vi "PI-Mono-Power.vi"() -> ()   [LabVIEW 2009]
uses:
  <vilib>/Utility/file.llb/Write To Spreadsheet File (DBL).vi
  <vilib>/Analysis/NI_AALBase.lvlib
  <vilib>/DAQmx/create/channels.llb/DAQmx Create Channel (AI-Voltage-Basic).vi
  <vilib>/DAQmx/configure/timing.llb/DAQmx Timing (Sample Clock).vi
  <vilib>/DAQmx/read.llb/DAQmx Read (Analog 1D DBL 1Chan NSamp).vi
  <vilib>/Utility/file.llb/Read From Spreadsheet File (DBL).vi
panel:
  in  "Open Power Normalization Values Path":path
  in  "Normalize with file?":bool
  in  "Power Values Path":path
  out "Normalized Current":cluster{dbl[], dbl[]}(graph)
  in  "Save Current Path":path
  in  "Save Current?":bool
  out "Spectral Current":cluster{dbl[], dbl[]}(graph)
  in  "End Scan":bool
  out "Measuring Current":bool
  in  "Current":tag
  in  "Current Scan":bool
  in  "Exit":bool
  out "Scanning":bool
  in  "Scan Save Path":path
  in  "Save Power Scan?":bool
  out "Power Scan":cluster{dbl[], dbl[]}(graph)
  in  "Abort\n Scan":bool
  in  "Wavelength\n   Step Size":dbl=1.0 min=0.1 max=100.0
  in  "Starting\nWavelength":dbl=400.0 min=400.0 max=2500.0
  in  "Ending\nWavelength":dbl=500.0 min=451.0 max=2501.0
  in  "Step Time (sec)":dbl=1.0 min=0.1 max=10.0 step=0.1
  in  "Measurement Save Path":path
  in  "Save Measurement?":bool
  out "Power Measurement":dbl[](graph)
  out "Readout value":dbl format="%^#_9e"
  out "Readout string":string
  in  "Timeout [ms]":i32=1000
  out "New":bool
  out "ZeroValue":dbl
  out "RANG_Val":dbl
  out "RANG_lbl":string
  out "Rng":string
  out "AUTO?":bool
  in  "AUTO":bool=TRUE
  in  "Range":i16=1 min=1 max=6 step=1
  out "PM Error log":string
  in  "Beam\nDiameter (mm)":dbl=4.0 min=1.0 max=9.0 step=0.5
  in  "BWIn":u16(ring) caption="Bandwidth" items=["HIGH", "LOW"]
  in  "Averaging Rate":i32=300 min=33 max=5000 step=1
  in  "Zero?":bool
  in  "Stop Measurement":bool
  out "Incrementing Down":bool
  out "Changing Wavelength":bool
  out "Incrementing Up":bool
  in  "Increment":dbl=10.0 min=0.1 max=50.0
  in  "Target\nWavelength":dbl=400.0 min=400.0 max=3000.0
  out "Wavelength (nm)":dbl
  out "Turning Turret":bool
  out "Current Blaze":string caption="Grating Blaze"
  out "Grating Density":dbl
  out "Grating Index":i32
  in  "Select Grating Blaze":string(combo)
  out "error out":errorcluster
  in  "Measure Power":bool
  in  "Switch Turret":bool
  in  "Scan":bool
  in  "Increment Down":bool
  in  "Increment Up":bool
  in  "Change Wavelength":bool
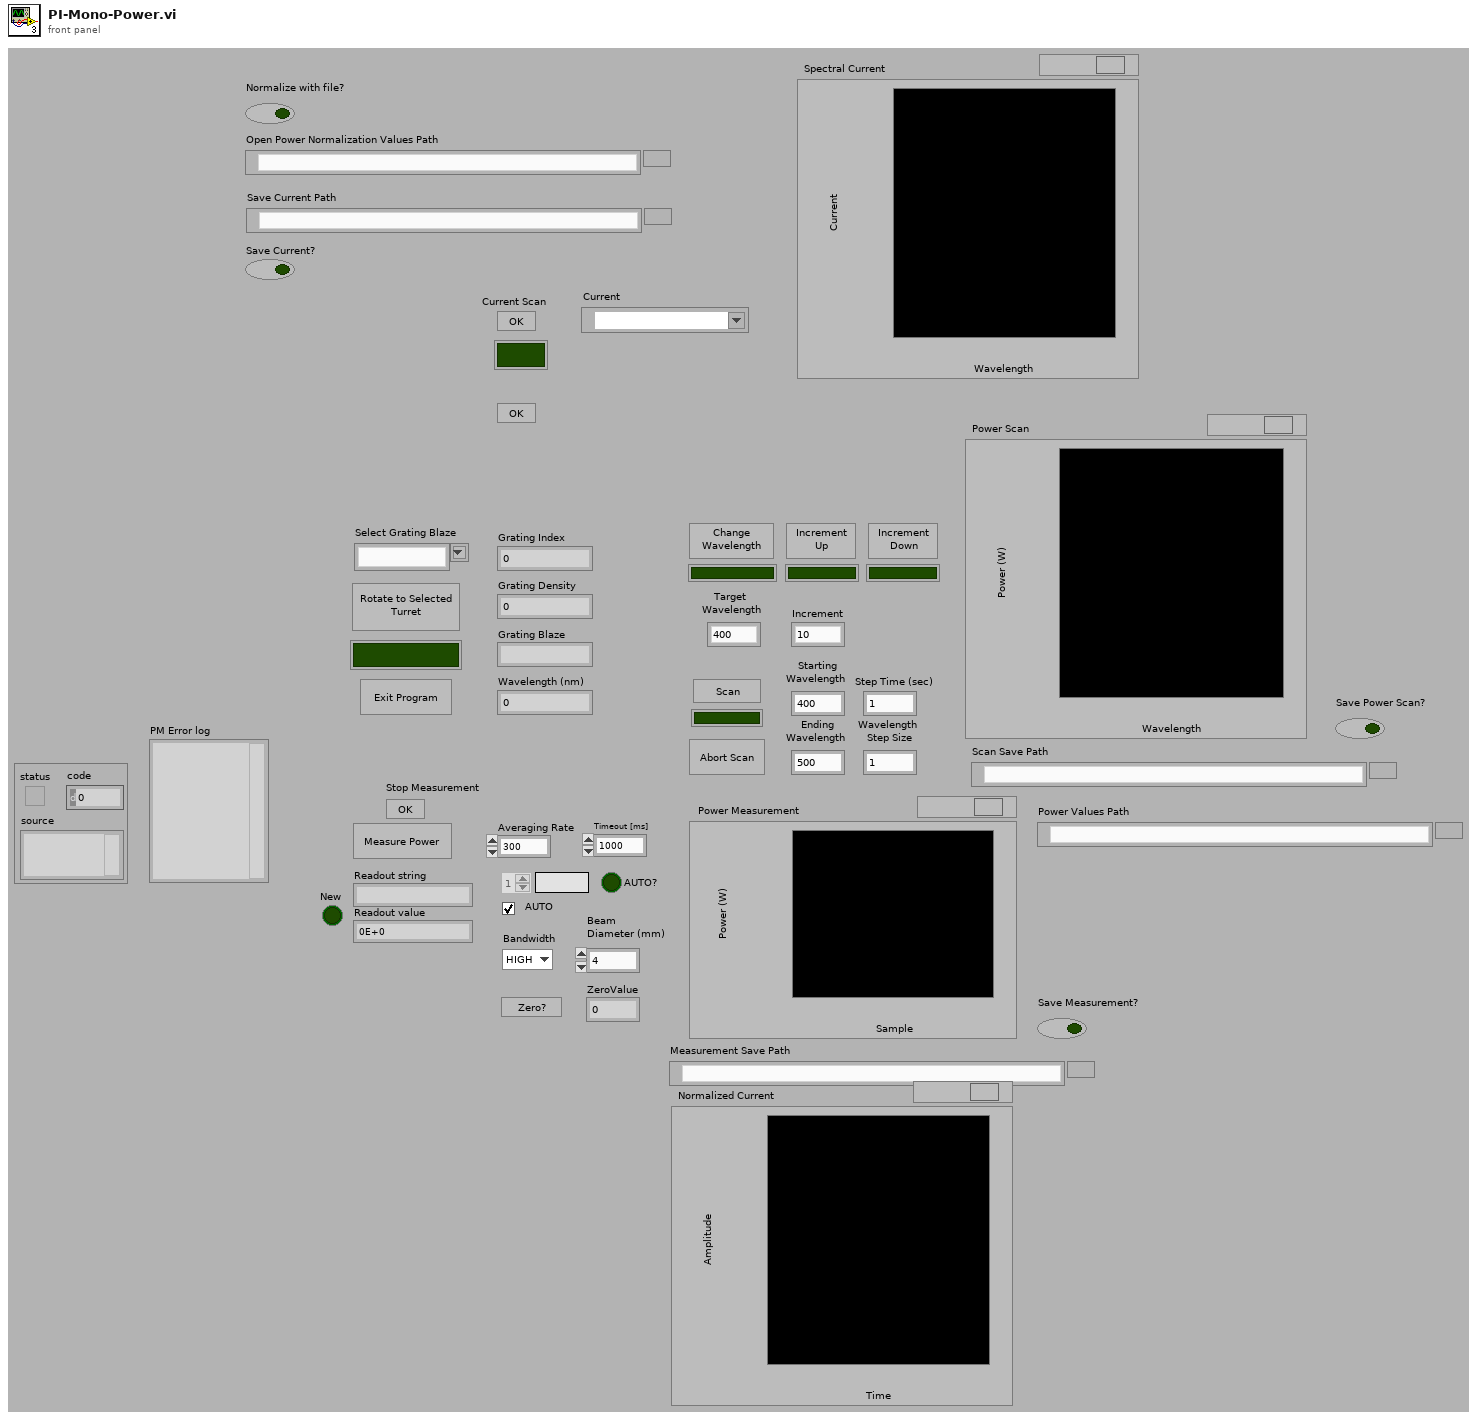
[diagram p1: front panel]
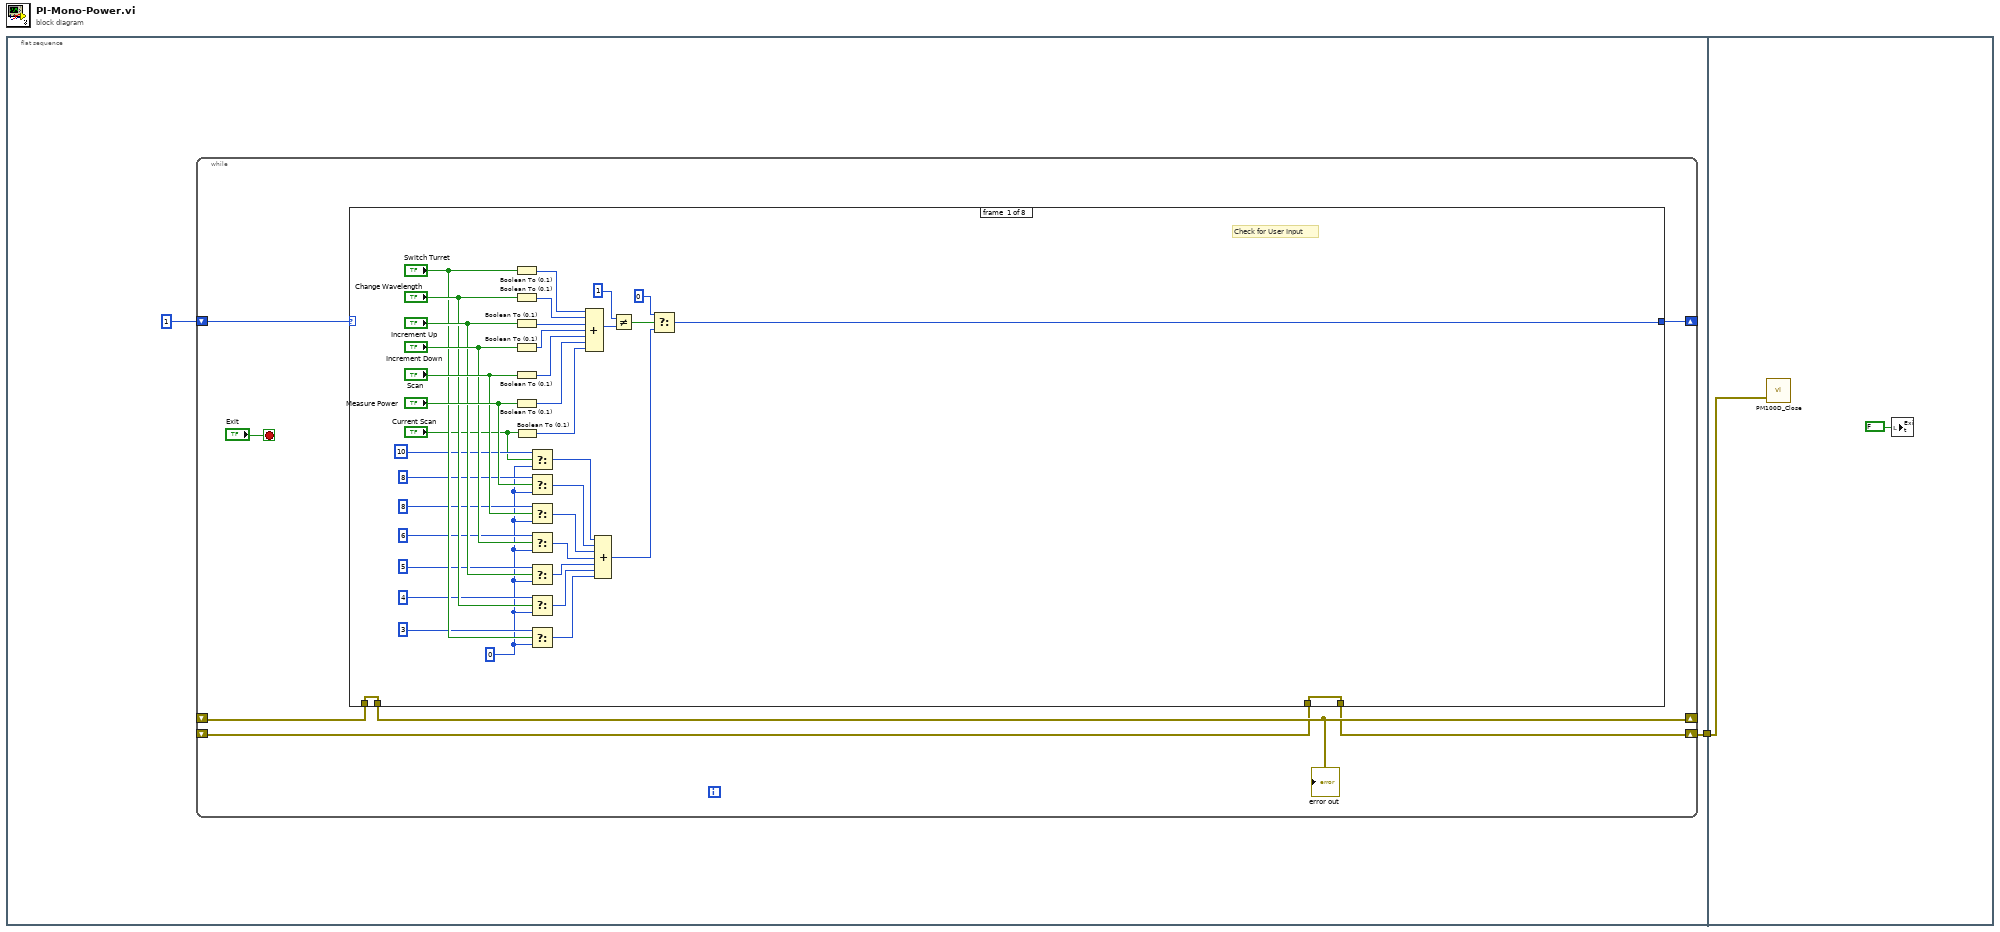
[diagram p0: block diagram]
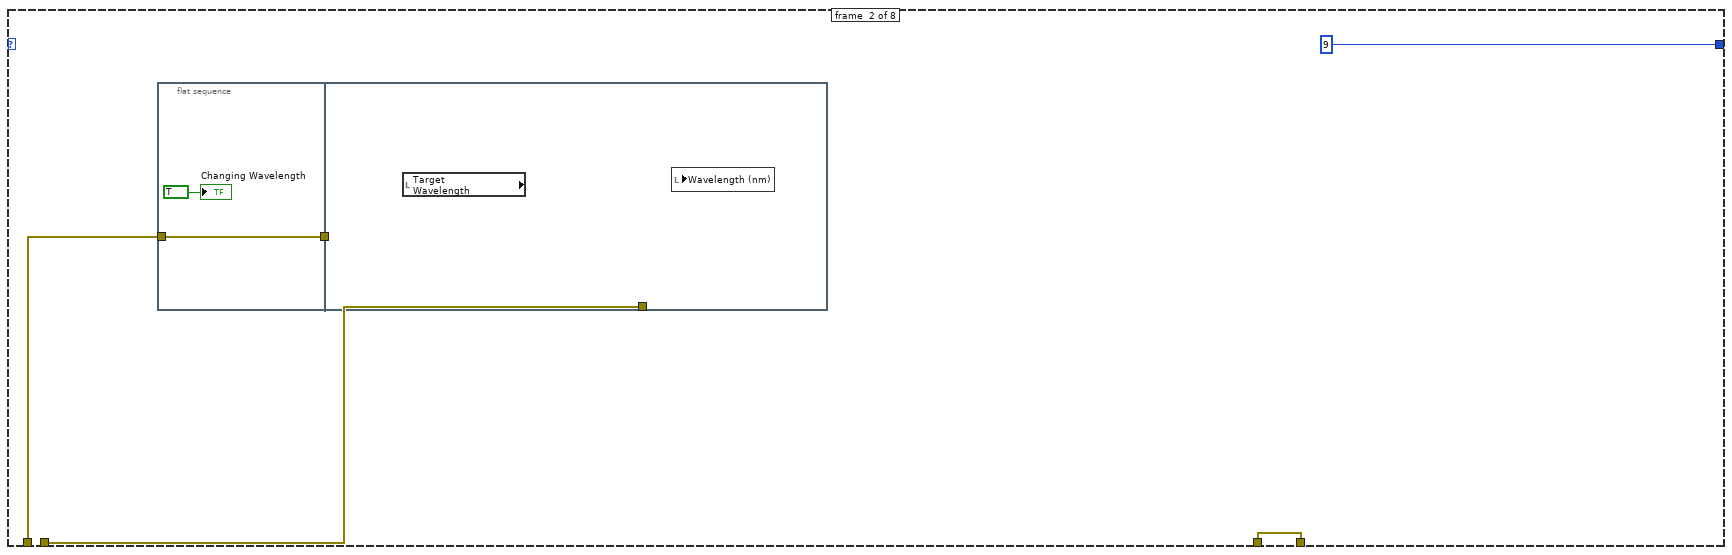
[diagram p2: hidden frame]
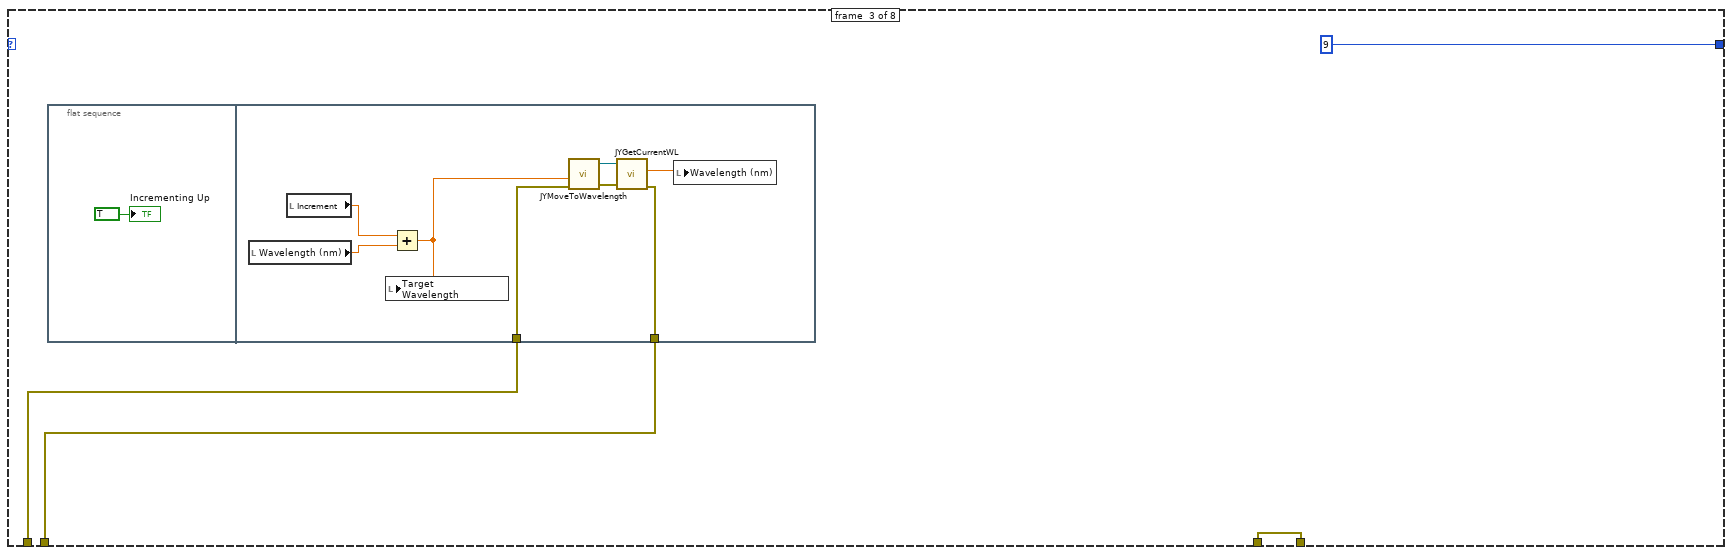
[diagram p3: hidden frame]
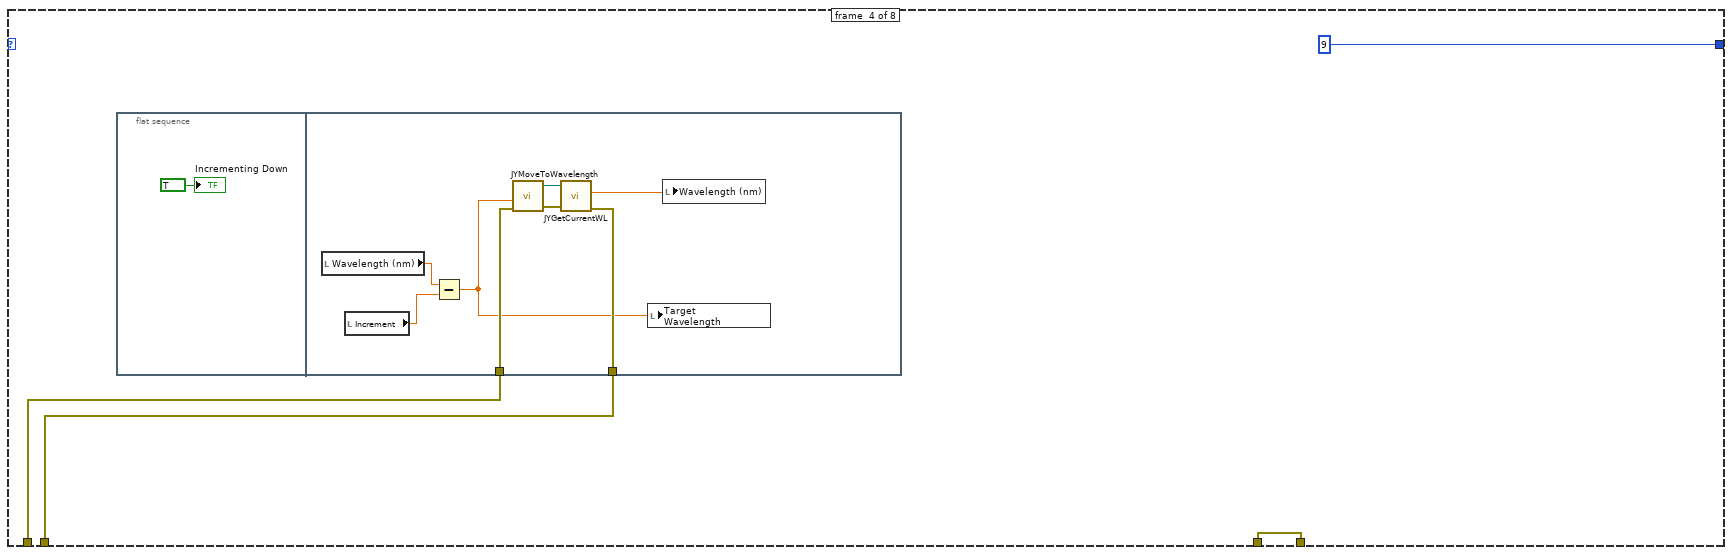
[diagram p4: hidden frame]
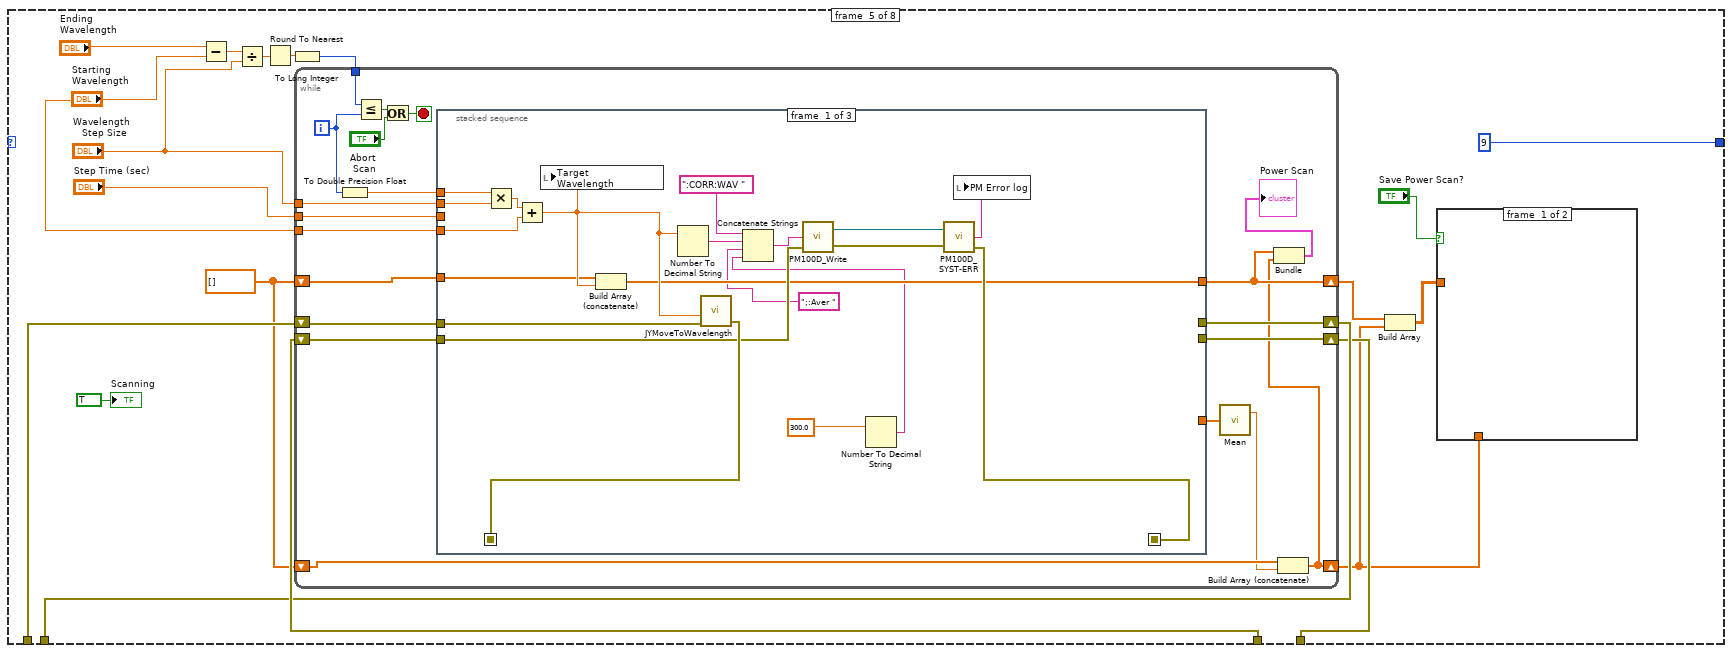
[diagram p5: hidden frame]
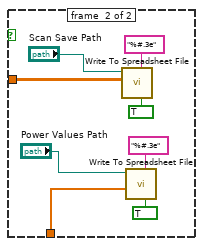
[diagram p6: hidden frame]
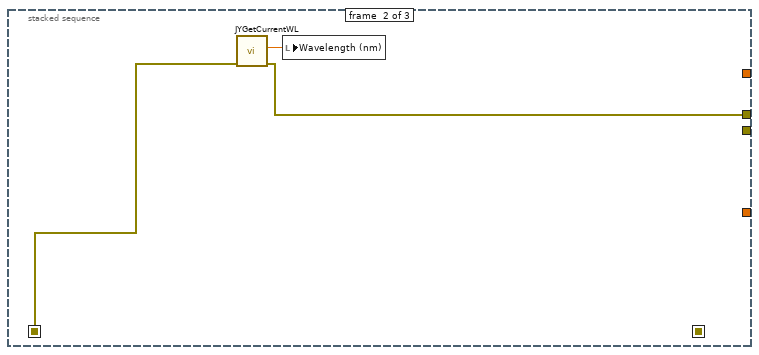
[diagram p7: hidden frame]
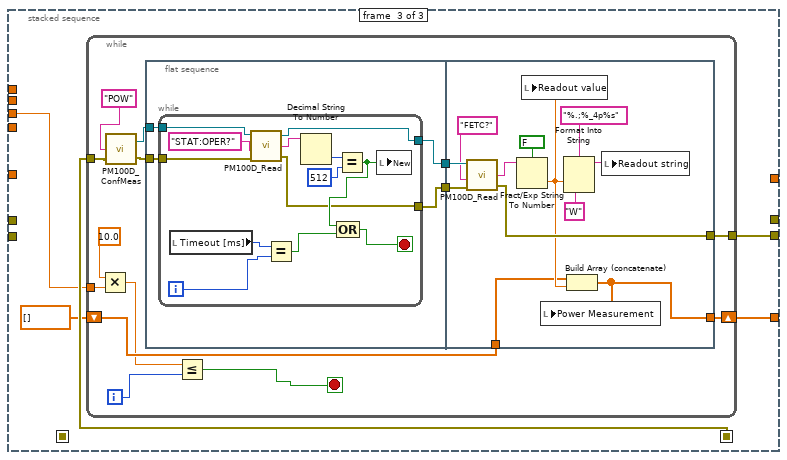
[diagram p8: hidden frame]
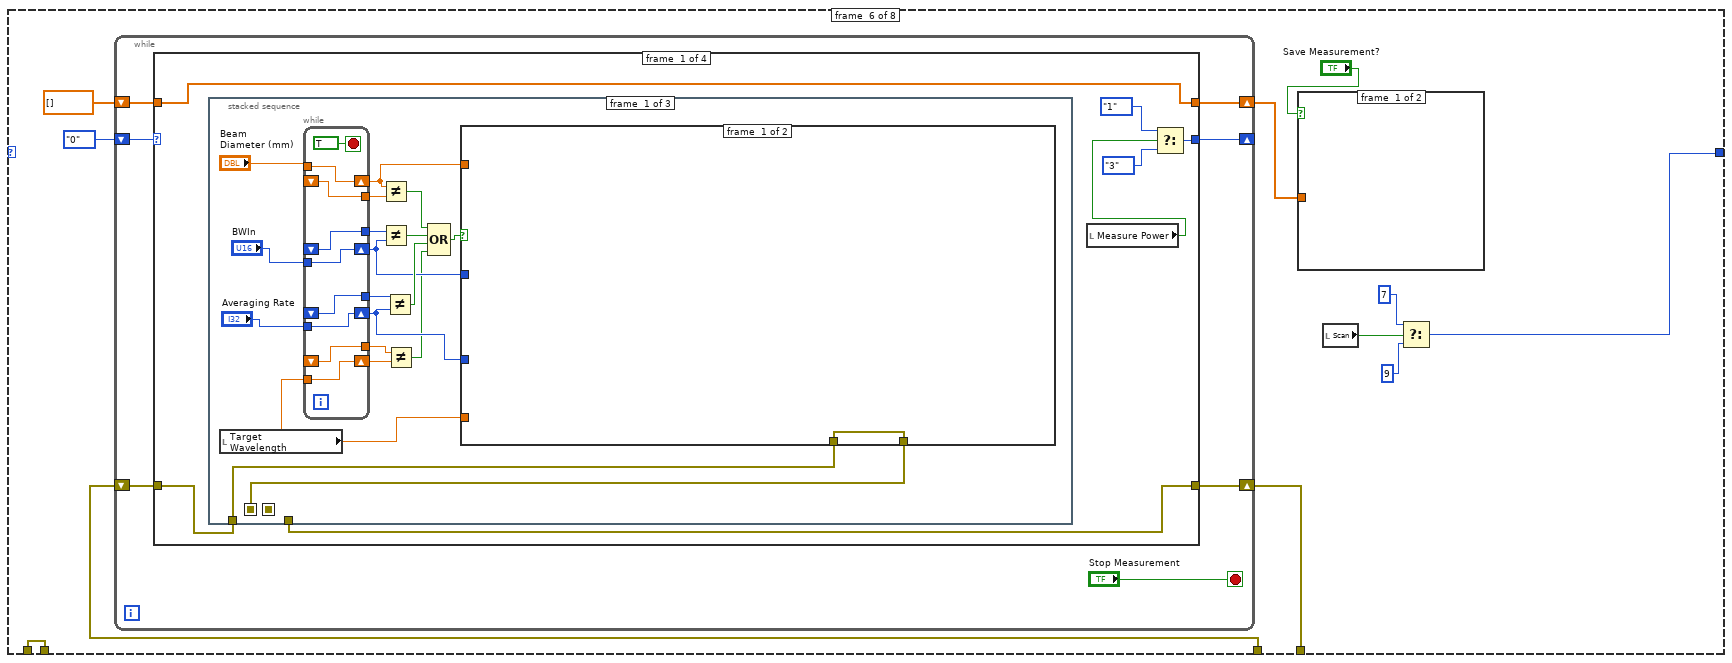
[diagram p9: hidden frame]
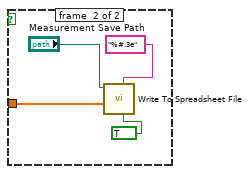
[diagram p10: hidden frame]
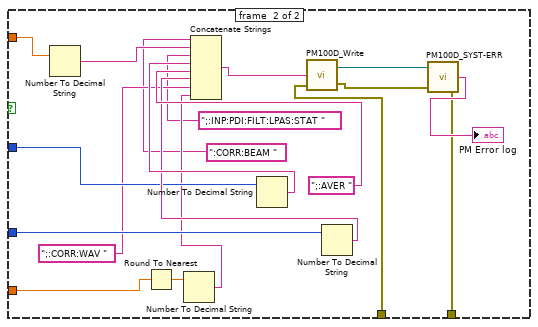
[diagram p11: hidden frame]
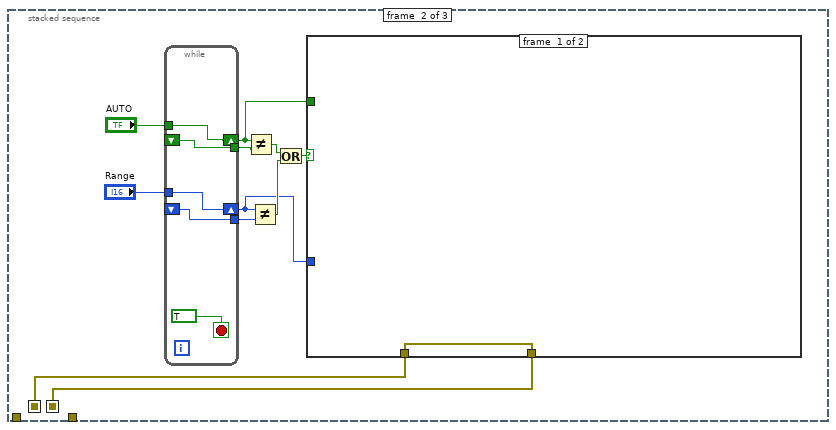
[diagram p12: hidden frame]
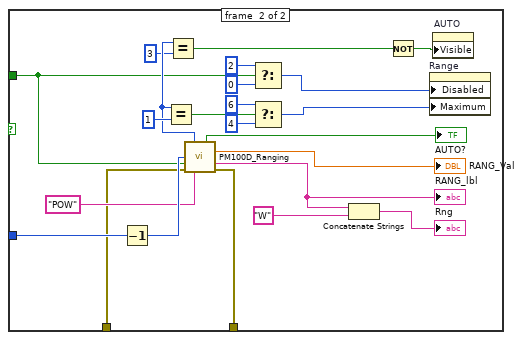
[diagram p13: hidden frame]
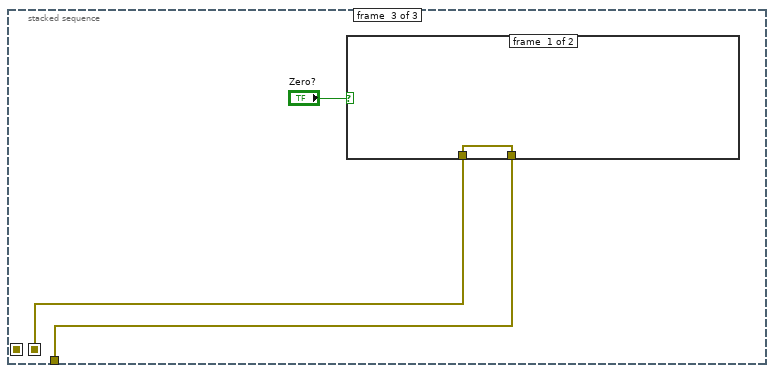
[diagram p14: hidden frame]
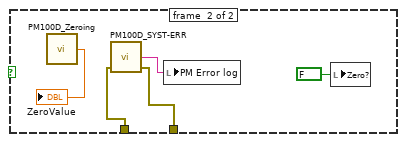
[diagram p15: hidden frame]
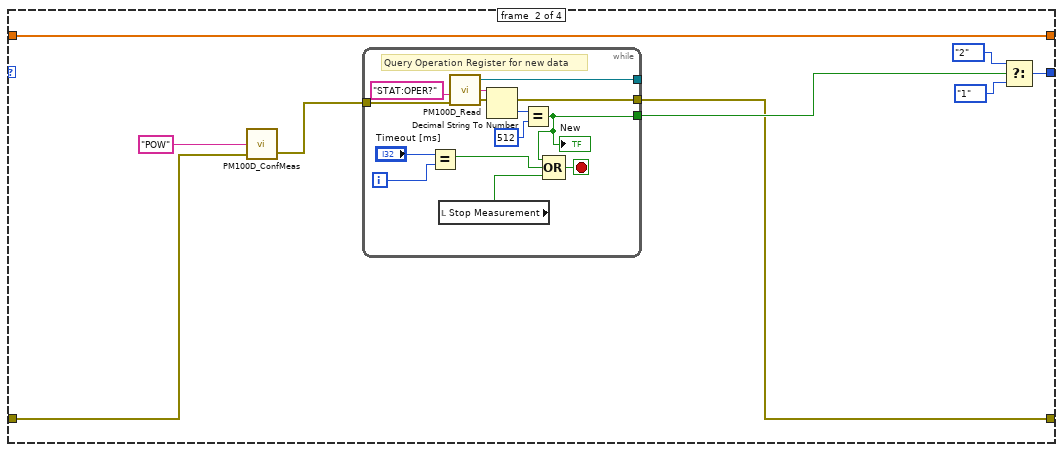
[diagram p16: hidden frame]
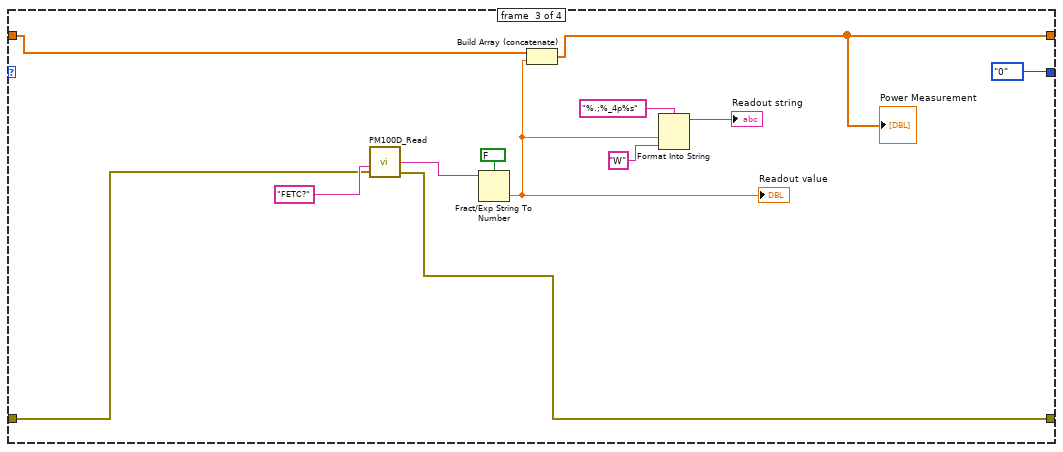
[diagram p17: hidden frame]
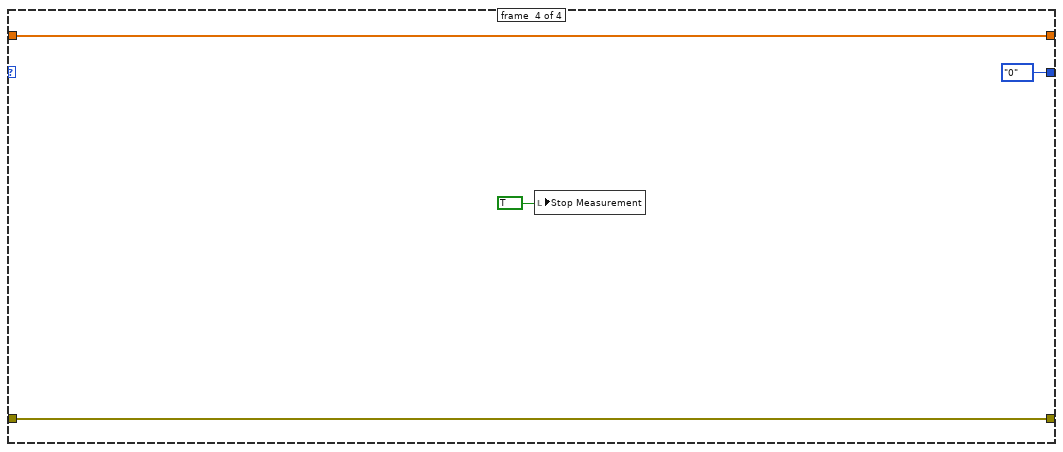
[diagram p18: hidden frame]
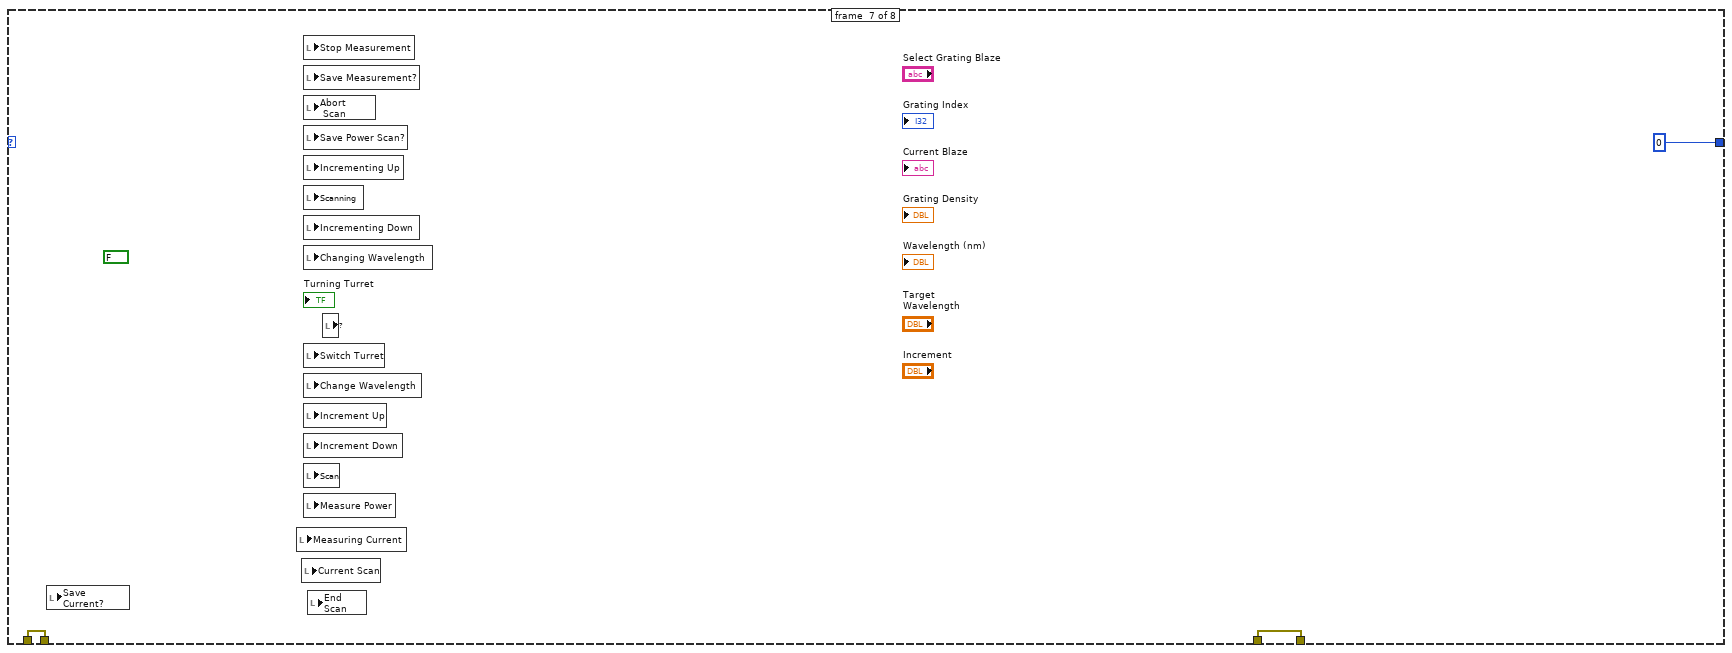
[diagram p19: hidden frame]
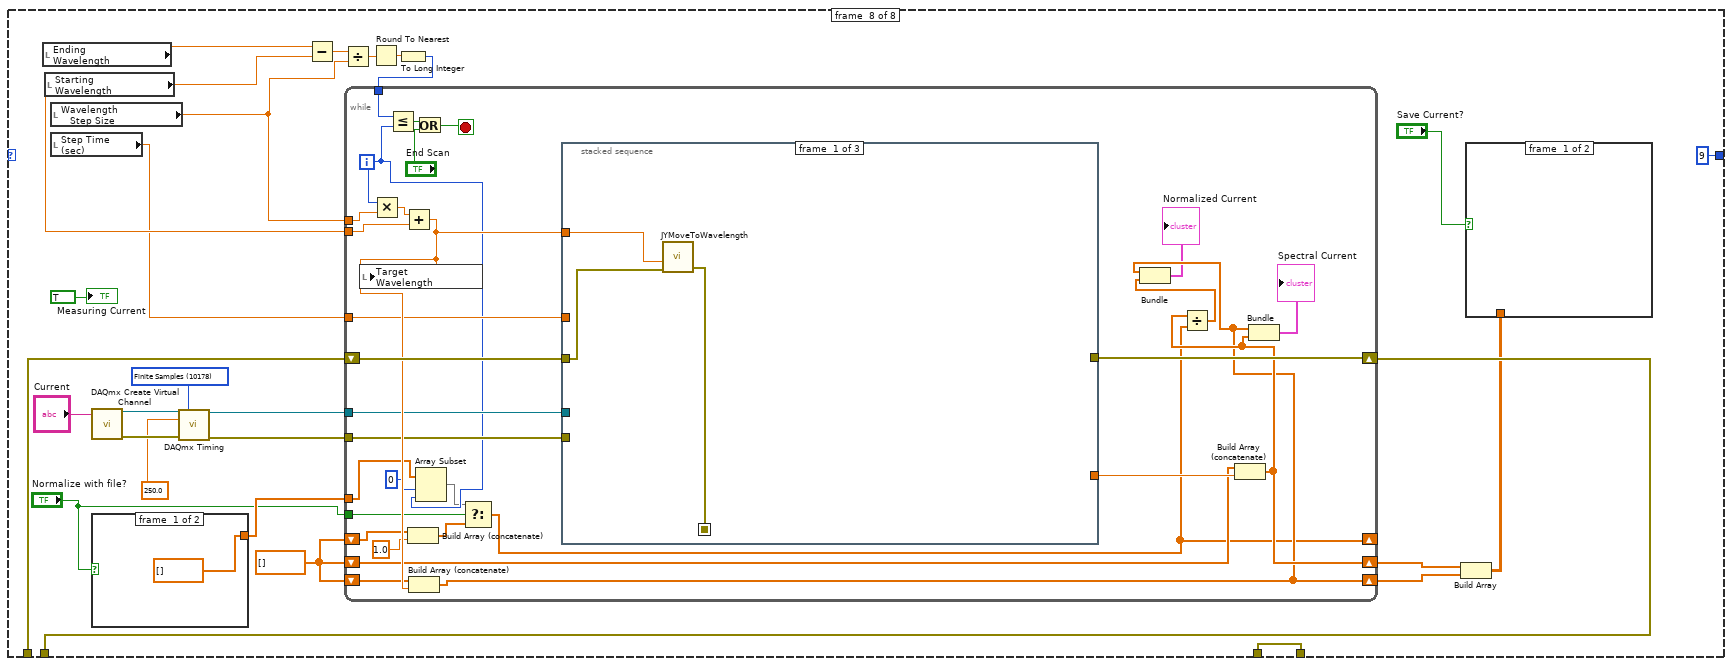
[diagram p20: hidden frame]
diagram:
  n1 = flat-sequence {
    tunnel: [w3] -> w1
    tunnel: w1 -> [w450]
    frame #0 {
      n2 = while {
        shift-right: [w10] -> _
        shift-left: 1 ("x") -> [w9]
        shift-right: [w7] -> _
        shift-left: _ -> [w8]
        shift-right: [w6] -> w3
        shift-left: _ -> [w5]
        stop <- "Exit" stop-if-true
        n3 = case shown="4" w9 {
          tunnel: [w19 9 ("x") 9 ("x") 9 ("x") 9 ("x") w199 0 ("x") 9 ("x")] -> w10
          tunnel: [w17 w50 w56 w70 w90 w209 w365 w382] -> w7
          tunnel: w8 -> [w17 w51 w57 w71 w92 w209 w365 w383]
          tunnel: [w16 w48 w55 w68 w89 w206 w364 w377] -> w6
          tunnel: w5 -> [w16 w48 w55 w68 w91 w207 w364 w377]
          frame #0 {
            w13 = 0 ("x")
            # "Check for User Input"
            n4 = Boolean To (0,1)(Boolean="Switch Turret") -> (0, 1=w47:i16)
            n5 = Boolean To (0,1)(Boolean="Change Wavelength") -> (0, 1=w46:i16)
            n6 = Boolean To (0,1)(Boolean="Increment Up") -> (0, 1=w45:i16)
            n7 = Boolean To (0,1)(Boolean="Increment Down") -> (0, 1=w44:i16)
            n8 = Boolean To (0,1)(Boolean="Scan") -> (0, 1=w43:i16)
            n9 = Boolean To (0,1)(Boolean="Measure Power") -> (0, 1=w42:i16)
            n10 = Boolean To (0,1)(Boolean="Current Scan") -> (0, 1=w15:i16)
            n11 = Select(t=10 ("x"), s="Current Scan", f=w13) -> (s? t:f=w14:i32)
            n12 = Select(t=8 ("x"), s="Measure Power", f=w13) -> (s? t:f=w33:i32)
            n13 = Select(t=8 ("x"), s="Scan", f=w13) -> (s? t:f=w32:i32)
            n14 = Select(t=6 ("x"), s="Increment Down", f=w13) -> (s? t:f=w31:i32)
            n15 = Select(t=5 ("x"), s="Increment Up", f=w13) -> (s? t:f=w30:i32)
            n16 = Select(t=4 ("x"), s="Change Wavelength", f=w13) -> (s? t:f=w29:i32)
            n17 = Select(t=3 ("x"), s="Switch Turret", f=w13) -> (s? t:f=w28:i32)
            n18 = Compound Arithmetic op=ADD(w47, w46, w45, w44, w43, w42, w15) -> (w41:i16)
            n19 = Compound Arithmetic op=ADD(w14, w33, w32, w31, w30, w29, w28) -> (w20:i32)
            n20 = Not Equal?(x=i16 1, y=w41) -> (x != y?=w27:bool)
            n21 = Select(t=0 ("x"), s=w27, f=w20) -> (s? t:f=w19:i32)
          }
          frame #1 {
            n22 = flat-sequence {
              tunnel: w51 -> [w54]
              tunnel: [w54] -> w49
              tunnel: [_] -> w50
              tunnel: w49 -> [_]
              frame #0 {
                "Changing Wavelength" <- TRUE
              }
              frame #1 {
                n23 = local read "Target\nWavelength"() -> ()  [unwired: 1 out]
                n24 = local read "Wavelength (nm)"() -> ()  [unwired: 1 in]
              }
            }
          }
          frame #2 {
            n25 = flat-sequence {
              tunnel: w57 -> [w65]
              tunnel: [w62] -> w56
              frame #0 {
                "Incrementing Up" <- TRUE
              }
              frame #1 {
                n26 = local read "Wavelength (nm)"() -> (w66:dbl)
                n27 = local read "Increment"() -> (w67:dbl)
                n28 = Add(x=w67, y=w66) -> (x+y=w61:dbl)
                n29 = local write "Target\nWavelength"(w61) -> ()
                n30 = call "JYMoveToWavelength.vi"("error in (no error)"=w65, "Target WL"=w61) -> ("error out"=w64:errorcluster, "Refnum Out"=w63:refnum<k7>)  [unwired: 2 in, 1 out]
                n31 = call "JYGetCurrentWL.vi"("error in (no error)"=w64, "JYMONOLib.IJYMonoReqd"=w63) -> ("error out"=w62:errorcluster, "Current WL"=w60:dbl)  [unwired: 6 in, 2 out]
                n32 = local write "Wavelength (nm)"(w60) -> ()
              }
            }
          }
          frame #3 {
            n33 = flat-sequence {
              tunnel: w71 -> [w76]
              tunnel: [w75] -> w70
              frame #0 {
                "Incrementing Down" <- TRUE
              }
              frame #1 {
                n34 = local read "Wavelength (nm)"() -> (w78:dbl)
                n35 = local read "Increment"() -> (w77:dbl)
                n36 = Subtract(x=w78, y=w77) -> (x-y=w74:dbl)
                n37 = call "JYMoveToWavelength.vi"("error in (no error)"=w76, "Target WL"=w74) -> ("error out"=w80:errorcluster, "Refnum Out"=w79:refnum<k7>)  [unwired: 2 in, 1 out]
                n38 = call "JYGetCurrentWL.vi"("error in (no error)"=w80, "JYMONOLib.IJYMonoReqd"=w79) -> ("error out"=w75:errorcluster, "Current WL"=w73:dbl)  [unwired: 6 in, 2 out]
                n39 = local write "Target\nWavelength"(w74) -> ()
                n40 = local write "Wavelength (nm)"(w73) -> ()
              }
            }
          }
          frame #4 {
            w88 = dbl[] []
            n41 = Subtract(x="Ending\nWavelength", y="Starting\nWavelength") -> (x-y=w97:dbl)
            n42 = Divide(x=w97, y="Wavelength\n   Step Size") -> (x/y=w83:dbl)
            n43 = Round To Nearest(number=w83) -> (nearest integer value=w82:dbl)
            n44 = To Long Integer(number=w82) -> (32bit integer=w96:i32)
            n45 = while {
              tunnel: w96 -> [w127]
              tunnel: "Wavelength\n   Step Size" -> [w123]
              tunnel: "Step Time (sec)" -> [w122]
              tunnel: "Starting\nWavelength" -> [w121]
              shift-right: [w110] -> w87
              shift-left: w88 -> [w116]
              shift-right: [w115] -> w90
              shift-left: w92 -> [w118]
              shift-right: [w114] -> w89
              shift-left: w91 -> [w117]
              shift-right: [w109] -> w81
              shift-left: w88 -> [w112]
              i -> [w120]
              stop <- w125 stop-if-true
              n46 = To Double Precision Float(number=w120) -> (double precision float=w119:dbl)
              n47 = Less Or Equal?(x=w127, y=w120) -> (x <= y?=w126:bool)
              n48 = Or(x=w126, y="Abort\n Scan") -> (x .or. y?=w125:bool)
              n49 = stacked-sequence {
                seq-local: [w138 _ _] -> [_ w150 _]
                seq-local: [w136 _ _] -> [_ _ w155]
                tunnel: w123 -> [w143 _ _]
                tunnel: w122 -> [_ _ w152]
                tunnel: w121 -> [w140 _ _]
                tunnel: w119 -> [w142 _ _]
                tunnel: w118 -> [w139 _ _]
                tunnel: w117 -> [w137 _ _]
                tunnel: w116 -> [w134 _ _]
                tunnel: [w133 _ _] -> w110
                tunnel: [_ w149 _] -> w115
                tunnel: [_ _ w154] -> w114
                tunnel: [_ _ w151] -> w113
                frame #0 {
                  n50 = Multiply(x=w142, y=w143) -> (x*y=w141:dbl)
                  n51 = Add(x=w141, y=w140) -> (x+y=w135:dbl)
                  n52 = local write "Target\nWavelength"(w135) -> ()
                  n53 = Build Array (concatenate)(w134, w135) -> (w133:dbl[])
                  n54 = Number To Decimal String(number=w135) -> (decimal integer string=w146:string)  [unwired: 1 in]
                  n55 = call "JYMoveToWavelength.vi"("error in (no error)"=w139, "Target WL"=w135) -> ("error out"=w138:errorcluster)  [unwired: 2 in, 2 out]
                  n56 = Number To Decimal String(number=300.0 ("y")) -> (decimal integer string=w130:string)  [unwired: 1 in]
                  n57 = Concatenate Strings(":CORR:WAV " ("string"), w146, ";:Aver " ("string"), w130) -> (w147:string)
                  n58 = call "PM100D_Write.vi"("error in (no error)"=w137, "Command"=w147) -> ("error out"=w131:errorcluster, "VISA out"=w132:refnum<visa-resource-name>)  [unwired: 1 in]
                  n59 = call "PM100D_SYST-ERR.vi"("error out 2"=w131, "VISA In"=w132) -> ("error out"=w136:errorcluster, "Error"=w144:string)  [unwired: 1 in, 1 out]
                  n60 = local write "PM Error log"(w144) -> ()
                }
                frame #1 {
                  n61 = call "JYGetCurrentWL.vi"("error in (no error)"=w150) -> ("error out"=w149:errorcluster, "Current WL"=w148:dbl)  [unwired: 7 in, 2 out]
                  n62 = local write "Wavelength (nm)"(w148) -> ()
                }
                frame #2 {
                  n63 = while {
                    tunnel: w155 -> [w169]
                    tunnel: [w163] -> w154
                    shift-right: [w161] -> w151
                    shift-left: dbl[] [] -> [w162]
                    tunnel: w152 -> [w159]
                    i -> [w160]
                    stop <- w156 stop-if-true
                    n64 = Multiply(x=10.0 ("y"), y=w159) -> (x*y=w157:dbl)
                    n65 = call "PM100D_ConfMeas.vi"("error in"=w169, "Conf:"="POW" ("Command")) -> ("error out"=w168:errorcluster, "dup VISA session"=w166:refnum<visa-resource-name>)  [unwired: 1 in]
                    n66 = flat-sequence {
                      tunnel: w168 -> [w173]
                      tunnel: w166 -> [w172]
                      tunnel: [w171] -> w165
                      tunnel: [w170] -> w164
                      tunnel: w165 -> [w195]
                      tunnel: w164 -> [w194]
                      tunnel: [w190] -> w163
                      tunnel: w162 -> [w188]
                      tunnel: [w187] -> w161
                      frame #0 {
                        n67 = while {
                          tunnel: w173 -> [w177]
                          tunnel: [w176] -> w170
                          tunnel: w172 -> [w175]
                          tunnel: [w174] -> w171
                          i -> [w185]
                          stop <- w186 stop-if-true
                          n68 = local read "Timeout [ms]"() -> (w184:i32)
                          n69 = call "PM100D_Read.vi"("error in (no error)"=w177, "Command"="STAT:OPER?", "VISA in"=w175) -> ("error out"=w176:errorcluster, "ReadValue"=w179:string, "VISA out"=w174:refnum<visa-resource-name>)  [unwired: 1 in]
                          n70 = Equal?(x=w184, y=w185) -> (x = y?=w183:bool)
                          n71 = Decimal String To Number(string=w179) -> (number=w182:i32)  [unwired: 2 in, 1 out]
                          n72 = Equal?(x=w182, y=512) -> (x = y?=w180:bool)
                          n73 = Compound Arithmetic op=OR(w180, w183) -> (w186:bool)
                          n74 = local write "New"(w180) -> ()
                        }
                      }
                      frame #1 {
                        n75 = call "PM100D_Read.vi"("error in (no error)"=w194, "Command"="FETC?", "VISA in"=w195) -> ("error out"=w190:errorcluster, "ReadValue"=w192:string)  [unwired: 1 in, 1 out]
                        n76 = Fract/Exp String To Number(use system decimal point (T)=FALSE, string=w192) -> (number=w189:dbl)  [unwired: 2 in, 1 out]
                        n77 = local write "Readout value"(w189) -> ()
                        n78 = Format Into String(format string="%.;%_4p%s", w189, "W") -> (resulting string=w191:string)  [unwired: 2 in, 1 out]
                        n79 = Build Array (concatenate)(w188, w189) -> (w187:dbl[])
                        n80 = local write "Power Measurement"(w187) -> ()
                        n81 = local write "Readout string"(w191) -> ()
                      }
                    }
                    n82 = Less Or Equal?(x=w157, y=w160) -> (x <= y?=w156:bool)
                  }
                }
              }
              n83 = call <vilib>:"Mean.vi"("X"=w113) -> ("mean"=w111:dbl)  [unwired: 1 out]
              n84 = Build Array (concatenate)(w112, w111) -> (w109:dbl[])
              n85 = Bundle(w110, w109) -> (→"Power Scan":cluster{dbl[], dbl[]})  [unwired: 1 in]
            }
            n86 = Build Array(w87, w81) -> (w86:dbl[][])
            n87 = case shown="True" "Save Power Scan?" {
              tunnel: w86 -> [_ w104]
              tunnel: w81 -> [_ w100]
              frame #0 {
              }
              frame #1 {
                n88 = call-poly <vilib>:"Write To Spreadsheet File.vi"("transpose? (no:F)"=TRUE, "format (%.3f)"="%#.3e", "2D data"=w104, "file path (dialog if empty)"="Scan Save Path") -> ()  [unwired: 4 in, 1 out]
                n89 = call-poly <vilib>:"Write To Spreadsheet File.vi"("transpose? (no:F)"=TRUE, "format (%.3f)"="%#.3e", "1D data"=w100, "file path (dialog if empty)"="Power Values Path") -> ()  [unwired: 4 in, 1 out]
              }
            }
            "Scanning" <- TRUE ("Scanning")
          }
          frame #5 {
            n90 = while {
              shift-right: [w219] -> _
              shift-left: enum16{"0", "1", "2", "3"}."0" -> [w220]
              shift-right: [w217] -> w206
              shift-left: w207 -> [w218]
              shift-right: [w215] -> w203
              shift-left: dbl[] [] -> [w216]
              stop <- "Stop Measurement" stop-if-true
              n91 = case shown="\"0\", Default" w220 {
                tunnel: [w224 w332 enum16{"0", "1", "2", "3"}."0" enum16{"0", "1", "2", "3"}."0"] -> w219
                tunnel: w218 -> [w227 w330 w353 w361]
                tunnel: [w226 w328 w352 w361] -> w217
                tunnel: w216 -> [w225 w327 w349 w362]
                tunnel: [w225 w327 w348 w362] -> w215
                frame #0 {
                  n92 = stacked-sequence {
                    seq-local: [w233 _ _] -> [_ w277 _]
                    seq-local: [_ w276 _] -> [_ _ w317]
                    tunnel: w227 -> [w234 _ _]
                    tunnel: [_ _ w316] -> w226
                    frame #0 {
                      n93 = local read "Target\nWavelength"() -> (w228:dbl)
                      n94 = while {
                        shift-right: [w274] -> w235
                        shift-left: _ -> [w273]
                        shift-right: [w270] -> w236
                        shift-left: _ -> [w269]
                        shift-right: [w272] -> w232
                        shift-left: _ -> [w271]
                        tunnel: "Beam\nDiameter (mm)" -> [w274]
                        tunnel: [w273] -> w246
                        tunnel: "Averaging Rate" -> [w272]
                        tunnel: [w271] -> w245
                        tunnel: "BWIn" -> [w270]
                        tunnel: [w269] -> w237
                        shift-right: [w268] -> w230
                        shift-left: _ -> [w267]
                        tunnel: w228 -> [w268]
                        tunnel: [w267] -> w231
                        stop <- TRUE stop-if-true
                      }
                      n95 = Not Equal?(x=w235, y=w246) -> (x != y?=w242:bool)
                      n96 = Not Equal?(x=w237, y=w236) -> (x != y?=w243:bool)
                      n97 = Not Equal?(x=w245, y=w232) -> (x != y?=w244:bool)
                      n98 = Not Equal?(x=w231, y=w230) -> (x != y?=w229:bool)
                      n99 = Compound Arithmetic op=OR(w242, w243, w244, w229) -> (w241:bool)
                      n100 = case shown="True" w241 {
                        tunnel: w232 -> [_ w258]
                        tunnel: w236 -> [_ w257]
                        tunnel: w235 -> [_ w256]
                        tunnel: w234 -> [w247 w255]
                        tunnel: [w247 w254] -> w233
                        tunnel: w228 -> [_ w250]
                        frame #0 {
                        }
                        frame #1 {
                          n101 = Number To Decimal String(number=w256) -> (decimal integer string=w259:string)  [unwired: 1 in]
                          n102 = Round To Nearest(number=w250) -> (nearest integer value=w253:dbl)
                          n103 = Number To Decimal String(number=w253) -> (decimal integer string=w251:string)  [unwired: 1 in]
                          n104 = Number To Decimal String(number=w257) -> (decimal integer string=w263:string)  [unwired: 1 in]
                          n105 = Number To Decimal String(number=w258) -> (decimal integer string=w260:string)  [unwired: 1 in]
                          n106 = Concatenate Strings(":CORR:BEAM " ("string"), w259, ";:INP:PDI:FILT:LPAS:STAT ", w263, ";:AVER " ("string"), w260, ";:CORR:WAV " ("string"), w251) -> (w266:string)
                          n107 = call "PM100D_Write.vi"("error in (no error)"=w255, "Command"=w266) -> ("error out"=w264:errorcluster, "VISA out"=w265:refnum<visa-resource-name>)  [unwired: 1 in]
                          n108 = call "PM100D_SYST-ERR.vi"("error out 2"=w264, "VISA In"=w265) -> ("error out"=w254:errorcluster, "Error"=→"PM Error log":string)  [unwired: 1 in, 1 out]
                        }
                      }
                    }
                    frame #1 {
                      n109 = while {
                        shift-right: [w313] -> w278
                        shift-left: _ -> [w312]
                        shift-right: [w315] -> w279
                        shift-left: _ -> [w314]
                        tunnel: "AUTO" -> [w315]
                        tunnel: [w314] -> w285
                        tunnel: "Range" -> [w313]
                        tunnel: [w312] -> w282
                        stop <- TRUE stop-if-true
                      }
                      n110 = Not Equal?(x=w279, y=w285) -> (x != y?=w284:bool)
                      n111 = Not Equal?(x=w278, y=w282) -> (x != y?=w281:bool)
                      n112 = Or(x=w284, y=w281) -> (x .or. y?=w280:bool)
                      n113 = case shown="False" w280 {
                        tunnel: w279 -> [_ w293]
                        tunnel: w278 -> [_ w292]
                        tunnel: [w287 w289] -> w276
                        tunnel: w277 -> [w287 w288]
                        frame #0 {
                        }
                        frame #1 {
                          n114 = Decrement(x=w292) -> (x-1=w300:i16)
                          n115 = call "PM100D_Ranging.vi"("Index"=w300, "AUTO"=w293, "error in (no error)"=w288, "Unit"="POW") -> ("SensType"=w299:i32, "AUTO?"=→"AUTO?":bool, "RANG_Val"=→"RANG_Val":dbl, "RANG_lbl"=w308:string, "error out"=w289:errorcluster)  [unwired: 4 in, 3 out]
                          "RANG_lbl" <- w308
                          n116 = Equal?(x=w299, y=1) -> (x = y?=w304:bool)
                          n117 = Equal?(x=w299, y=3) -> (x = y?=w294:bool)
                          n118 = Select(t=2, s=w293, f=0) -> (s? t:f=w306:i32)
                          n119 = Select(t=6, s=w304, f=4) -> (s? t:f=w305:i32)
                          n120 = Concatenate Strings(w308, "W") -> (→"Rng":string)
                          n121 = Not(x=w294) -> (.not. x?=w295:bool)
                          n122 = property on="Range" class="DigNum (strict)"("Disabled"=w306, "Maximum"=w305) -> ()  [unwired: 2 in, 2 out]
                          n123 = property on="AUTO" class="Bool (strict)"("Visible"=w295) -> ()  [unwired: 2 in, 2 out]
                        }
                      }
                    }
                    frame #2 {
                      n124 = case shown="False" "Zero?" {
                        tunnel: w317 -> [w319 w323]
                        tunnel: [w319 w322] -> w316
                        frame #0 {
                        }
                        frame #1 {
                          n125 = call "PM100D_Zeroing.vi"() -> ("ZeroValue"=→"ZeroValue":dbl)  [unwired: 5 in]
                          n126 = call "PM100D_SYST-ERR.vi"("error out 2"=w323) -> ("error out"=w322:errorcluster, "Error"=w321:string)  [unwired: 2 in, 1 out]
                          n127 = local write "PM Error log"(w321) -> ()
                          n128 = local write "Zero?"(FALSE ("Zero?")) -> ()
                        }
                      }
                    }
                  }
                  n129 = local read "Measure Power"() -> (w223:bool)
                  n130 = Select(t=enum16{"0", "1", "2", "3"}."1", s=w223, f=enum16{"0", "1", "2", "3"}."3") -> (s? t:f=w224:enum16{"0", "1", "2", "3"})
                }
                frame #1 {
                  n131 = call "PM100D_ConfMeas.vi"("error in"=w330, "Conf:"="POW" ("Command")) -> ("error out"=w329:errorcluster)  [unwired: 1 in, 1 out]
                  n132 = while {
                    tunnel: w329 -> [w342]
                    tunnel: [w341] -> _
                    tunnel: [w340] -> w328
                    tunnel: [w335] -> w331
                    i -> [w337]
                    stop <- w339 stop-if-true
                    # "Query Operation Register for new data"
                    n133 = Equal?(x="Timeout [ms]", y=w337) -> (x = y?=w336:bool)
                    n134 = local read "Stop Measurement"() -> (w334:bool)
                    n135 = call "PM100D_Read.vi"("error in (no error)"=w342, "Command"="STAT:OPER?") -> ("error out"=w340:errorcluster, "ReadValue"=w345:string, "VISA out"=w341:refnum<visa-resource-name>)  [unwired: 2 in]
                    n136 = Decimal String To Number(string=w345) -> (number=w344:i32)  [unwired: 2 in, 1 out]
                    n137 = Equal?(x=w344, y=512) -> (x = y?=w335:bool)
                    "New" <- w335
                    n138 = Compound Arithmetic op=OR(w335, w336, w334) -> (w339:bool)
                  }
                  n139 = Select(t=enum16{"0", "1", "2", "3"}."2", s=w331, f=enum16{"0", "1", "2", "3"}."1") -> (s? t:f=w332:enum16{"0", "1", "2", "3"})
                }
                frame #2 {
                  n140 = call "PM100D_Read.vi"("error in (no error)"=w353, "Command"="FETC?") -> ("error out"=w352:errorcluster, "ReadValue"=w357:string)  [unwired: 2 in, 1 out]
                  n141 = Fract/Exp String To Number(use system decimal point (T)=FALSE, string=w357) -> (number=w350:dbl)  [unwired: 2 in, 1 out]
                  "Readout value" <- w350
                  n142 = Build Array (concatenate)(w349, w350) -> (w348:dbl[])
                  "Power Measurement" <- w348
                  n143 = Format Into String(format string="%.;%_4p%s", w350, "W" ("Command")) -> (resulting string=→"Readout string":string)  [unwired: 2 in, 1 out]
                }
                frame #3 {
                  n144 = local write "Stop Measurement"(TRUE ("t")) -> ()
                }
              }
            }
            n145 = case shown="False" "Save Measurement?" {
              tunnel: w203 -> [_ w210]
              frame #0 {
              }
              frame #1 {
                n146 = call-poly <vilib>:"Write To Spreadsheet File.vi"("transpose? (no:F)"=TRUE, "format (%.3f)"="%#.3e", "1D data"=w210, "file path (dialog if empty)"="Measurement Save Path") -> ()  [unwired: 4 in, 1 out]
              }
            }
            n147 = local read "Scan"() -> (w200:bool)
            n148 = Select(t=7 ("x"), s=w200, f=9 ("x")) -> (s? t:f=w199:i32)
          }
          frame #6 {
            (unwired) FALSE
            n149 = local read "Save Current?"() -> ()  [unwired: 1 in]
            n150 = local read "Measuring Current"() -> ()  [unwired: 1 in]
            n151 = local read "Current Scan"() -> ()  [unwired: 1 in]
            n152 = local read "Stop Measurement"() -> ()  [unwired: 1 in]
            n153 = local read "Save Measurement?"() -> ()  [unwired: 1 in]
            n154 = local read "Abort\n Scan"() -> ()  [unwired: 1 in]
            n155 = local read "Save Power Scan?"() -> ()  [unwired: 1 in]
            n156 = local read "Incrementing Up"() -> ()  [unwired: 1 in]
            n157 = local read "Scanning"() -> ()  [unwired: 1 in]
            n158 = local read "Incrementing Down"() -> ()  [unwired: 1 in]
            n159 = local read "Changing Wavelength"() -> ()  [unwired: 1 in]
            n160 = local read "Switch Turret"() -> ()  [unwired: 1 in]
            n161 = local read "Change Wavelength"() -> ()  [unwired: 1 in]
            n162 = local read "Increment Up"() -> ()  [unwired: 1 in]
            n163 = local read "Increment Down"() -> ()  [unwired: 1 in]
            n164 = local read "Scan"() -> ()  [unwired: 1 in]
            n165 = local read "Measure Power"() -> ()  [unwired: 1 in]
            n166 = local read "End Scan"() -> ()  [unwired: 1 in]
            n167 = local read item#-1() -> ()  [unwired: 1 in]
          }
          frame #7 {
            w378 = 10178 items=["Finite Samples"=10178, "Continuous Samples"=10123, "Hardware Timed Single Point"=12522] ("sample mode")
            w366 = dbl[] []
            n168 = local read "Ending\nWavelength"() -> (w387:dbl)
            n169 = local read "Starting\nWavelength"() -> (w385:dbl)
            n170 = local read "Wavelength\n   Step Size"() -> (w384:dbl)
            n171 = local read "Step Time (sec)"() -> (w371:dbl)
            n172 = call-poly <vilib>:"DAQmx Create Virtual Channel.vi"("physical channels"="Current") -> ("task out"=w380:refnum<k21>, "error out"=w381:errorcluster)  [unwired: 13 in]
            n173 = case shown="False" "Normalize with file?" {
              tunnel: [dbl[] [] w394] -> w368
              frame #0 {
              }
              frame #1 {
                n174 = call-poly <vilib>:"Read From Spreadsheet File.vi"("transpose (no:F)"=TRUE ("transpose? (no:F)"), "format (%.3f)"="%#.3e", "file path (dialog if empty)"="Open Power Normalization Values Path") -> ("first row"=w394:dbl[])  [unwired: 4 in, 4 out]
              }
            }
            n175 = call-poly <vilib>:"DAQmx Timing.vi"("task/channels in"=w380, "sample mode"=w378, "rate"=250.0, "error in"=w381) -> ("task out"=w370:refnum<k21>, "error out"=w369:errorcluster)  [unwired: 10 in]
            n176 = Subtract(x=w387, y=w385) -> (x-y=w390:dbl)
            n177 = Divide(x=w390, y=w384) -> (x/y=w389:dbl)
            n178 = Round To Nearest(number=w389) -> (nearest integer value=w388:dbl)
            n179 = To Long Integer(number=w388) -> (32bit integer=w386:i32)
            n180 = while {
              tunnel: w386 -> [w428]
              shift-right: [w414] -> w374
              shift-left: w366 -> [w418]
              tunnel: w385 -> [w425]
              tunnel: w384 -> [w427]
              shift-right: [w423] -> w382
              shift-left: w383 -> [w424]
              shift-right: [w412] -> w373
              shift-left: w366 -> [w419]
              tunnel: w370 -> [w421]
              tunnel: w371 -> [w416]
              tunnel: w369 -> [w415]
              tunnel: w368 -> [w408]
              tunnel: "Normalize with file?" -> [w410]
              shift-right: [w402] -> _
              shift-left: w366 -> [w404]
              i -> [w407]
              stop <- w431 stop-if-true
              n181 = Multiply(x=w407, y=w427) -> (x*y=w426:dbl)
              n182 = Less Or Equal?(x=w428, y=w407) -> (x <= y?=w430:bool)
              n183 = Add(x=w426, y=w425) -> (x+y=w422:dbl)
              n184 = local write "Target\nWavelength"(w422) -> ()
              n185 = Build Array (concatenate)(w404, 1.0 ("element")) -> (w403:dbl[])
              n186 = Build Array (concatenate)(w419, w422) -> (w412:dbl[])
              n187 = Or(x=w430, y="End Scan") -> (x .or. y?=w431:bool)
              n188 = Array Subset(array=w408, index=0, length=w407) -> (w406:dbl[])
              n189 = Select(t=w406, s=w410, f=w403) -> (s? t:f=w402:dbl[])
              n190 = stacked-sequence {
                seq-local: [w432 _ _] -> [_ w436 _]
                tunnel: w422 -> [w434 _ _]
                tunnel: w424 -> [w433 _ _]
                tunnel: [_ w435 _] -> w423
                tunnel: w421 -> [_ _ w449]
                tunnel: [_ _ w446] -> w420
                tunnel: w416 -> [_ _ w444]
                tunnel: w415 -> [_ _ w438]
                frame #0 {
                  n191 = call "JYMoveToWavelength.vi"("error in (no error)"=w433, "Target WL"=w434) -> ("error out"=w432:errorcluster)  [unwired: 2 in, 2 out]
                }
                frame #1 {
                  n192 = call "JYGetCurrentWL.vi"("error in (no error)"=w436) -> ("error out"=w435:errorcluster, "Current WL"=w437:dbl)  [unwired: 7 in, 2 out]
                  n193 = local write "Wavelength (nm)"(w437) -> ()
                }
                frame #2 {
                  n194 = Round To Nearest(number=w444) -> (nearest integer value=w445:dbl)
                  n195 = To Long Integer(number=w445) -> (32bit integer=w442:i32)
                  n196 = Multiply(x=250 ("number of samples per channel"), y=w442) -> (x*y=w441:i32)
                  n197 = call-poly <vilib>:"DAQmx Read.vi"("task/channels in"=w449, "number of samples per channel"=w441, "timeout"=10.0, "error in"=w438) -> ("task out"=w439:refnum<k21>, "data"=w447:dbl[], "error out"=w440:errorcluster)  [unwired: 9 in]
                  n198 = call <vilib>:"DAQmx Stop Task.vi"("task/channels in"=w439, "error in"=w440) -> ()  [unwired: 12 in, 2 out]
                  n199 = call <vilib>:"Mean.vi"("X"=w447) -> ("mean"=w446:dbl)  [unwired: 1 out]
                }
              }
              n200 = Build Array (concatenate)(w418, w420) -> (w414:dbl[])
              n201 = Divide(x=w414, y=w402) -> (x/y=w413:dbl[])
              n202 = Bundle(w412, w413) -> (→"Normalized Current":cluster{dbl[], dbl[]})  [unwired: 1 in]
              n203 = Bundle(w412, w414) -> (→"Spectral Current":cluster{dbl[], dbl[]})  [unwired: 1 in]
            }
            n204 = Build Array(w374, w373) -> (w372:dbl[][])
            n205 = case shown="True" "Save Current?" {
              tunnel: w372 -> [_ w398]
              frame #0 {
              }
              frame #1 {
                n206 = call-poly <vilib>:"Write To Spreadsheet File.vi"("transpose? (no:F)"=TRUE, "format (%.3f)"="%#.3e", "2D data"=w398, "file path (dialog if empty)"="Save Current Path") -> ()  [unwired: 4 in, 1 out]
              }
            }
            "Measuring Current" <- TRUE ("Scanning")
          }
        }
        "error out" <- w7
      }
    }
    frame #1 {
      n207 = call "PM100D_Close.vi"("error in (no error)"=w450) -> ()  [unwired: 3 in]
      n208 = local write "Exit"(FALSE ("Exit")) -> ()
    }
  }
